vi "Shutdown.vi"(8 "error in (no error)":errorcluster, 11 "Type Converter in":refnum<class "String Type Buffer Converter.lvclass">) -> (0 "error out":errorcluster, 3 "Type Converter out":refnum<class "String Type Buffer Converter.lvclass">)   [LabVIEW 2017, in "String Type Buffer Converter.lvlib" / "String Type Buffer Converter.lvclass"]
uses:
  String Type Buffer Converter.lvclass
  String Type Buffer Converter.lvclass/String Type Buffer Converter.ctl
  Conversion.ctl
  Conversion Block.ctl
  Builds/Data Sharing Framework/Current/Data Sharing Framework Core/DSF Core.lvlibp/Engine/Classes/Buffer Converter/Channel Descriptor.ctl
  Builds/Data Sharing Framework/Current/Data Sharing Framework Core/DSF Core.lvlibp/DSF Configuration API/Public/Controls/DSF Data Type.ctl
  Builds/Data Sharing Framework/Current/Data Sharing Framework Core/DSF Core.lvlibp
  Builds/Data Sharing Framework/Current/Data Sharing Framework Core/DSF Core.lvlibp/Engine/Classes/Buffer/Buffer.lvclass
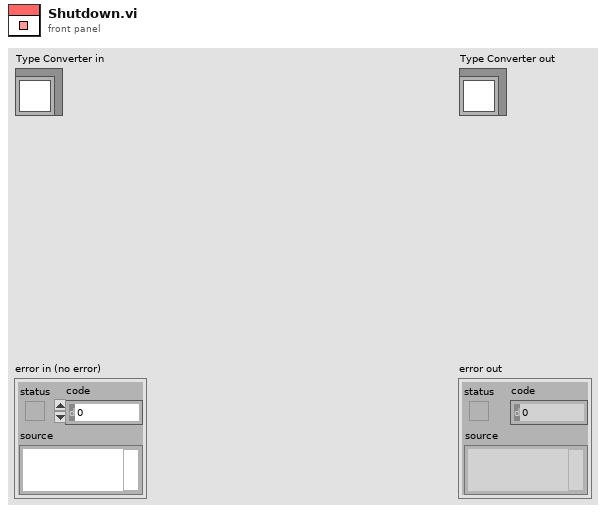
[diagram p1: front panel]
types:
  T1 = typedef "String Type Buffer Converter.lvlib/String Type Buffer Converter.lvclass/Conversion.ctl" = cluster{"conversion blocks":T2[]}
  T2 = typedef "String Type Buffer Converter.lvlib/String Type Buffer Converter.lvclass/Conversion Block.ctl" = cluster{"engine block descriptor":T3, "string block descriptor":T3, "engine byte order":enum16{"big-endian, network order", "native, host order", "little-endian"}, "string byte order":enum16{"big-endian, network order", "native, host order", "little-endian"}, "count":u64}
  T3 = typedef "DSF Core.lvlibp/Buffer.lvclass/Channel Descriptor.ctl" = cluster{"buffer offset":u64, "data type":T4}
  T4 = typedef "DSF Core.lvlibp/DSF Data Type.ctl" = enum8{"Bool", "SGL", "DBL", "I8", "I16", "I32", "I64", "U8", "U16", "U32", "U64"}
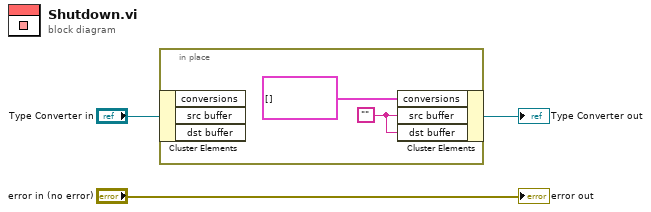
[diagram p0: block diagram]
diagram:
  n1 = in-place {
    w4 = ""
    n2 = in-place-cluster #1("Type Converter in") -> ()  [unwired: 3 out]
    n3 = in-place-cluster #1("conversions"=T1[] [], "src buffer"=w4, "dst buffer"=w4) -> (→"Type Converter out":refnum<class "String Type Buffer Converter.lvclass">)
  }
  "error out" <- "error in (no error)"
